vi "Configure Hardware.vi"(8 "error in (no error)":T3 caption="entrée d'erreur (pas d'erreur)", 11 "Ressources matérielles en entrée":T1) -> (0 "error out":T3 caption="sortie d'erreur", 3 "Ressources matérielles en sortie":T1)   [LabVIEW 2020, in "Acquisition.lvlib"]
doc: "Configurez le matériel."
uses:
  Acquisition.lvlib
  Hardware Configuration.ctl
  Signal Type.ctl
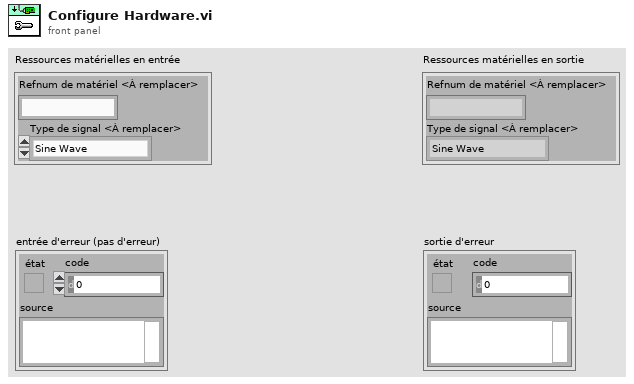
[diagram p1: front panel]
types:
  T1 = typedef "Acquisition.lvlib/Hardware Configuration.ctl" = cluster{"Refnum de matériel <À remplacer>":string, "Type de signal <À remplacer>":T2}
  T2 = typedef "Acquisition.lvlib/Signal Type.ctl" = enum16{"Sine Wave", "Square with Noise", "Signal triangulaire", "Simulation DAQ"}
  T3 = cluster{"état":bool, "code":i32, "source":string}
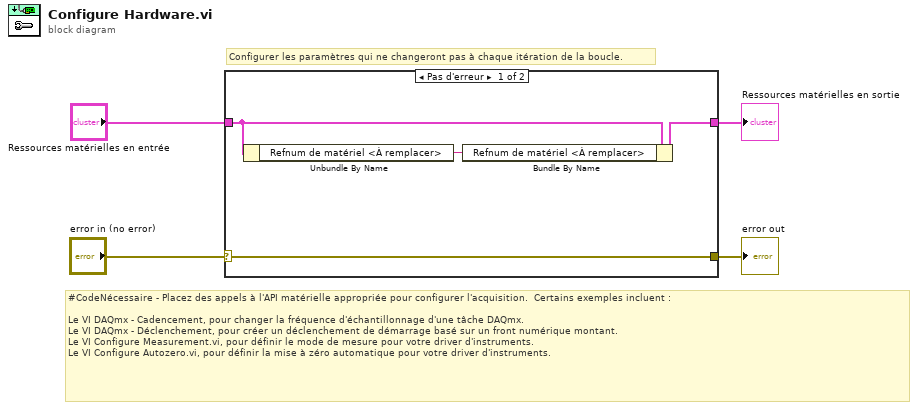
[diagram p0: block diagram]
diagram:
  # "Configurer les paramètres qui ne changeront pas à chaque itération de la boucle."
  # "#CodeNécessaire - Placez des appels à l'API matérielle appropriée pour configurer l'acquisition.  Certains exemples incluent :\n\nLe VI DAQmx - Cadencement, pour changer la fréquence d'échantillonnage d'une tâche DAQmx.\nLe VI DAQmx - Déclenchement, pour créer un déclenchement de démarrage basé sur un front numérique montant.\nLe VI Configure Measurement.vi, pour définir le mode de mesure pour votre driver d'instruments.\nLe VI Configure Autozero.vi, pour définir la mise à zéro automatique pour votre driver d'instruments."
  n1 = case shown="Pas d'erreur" "error in (no error)" {
    selector: "error in (no error)" -> [w7 w9]
    tunnel: [w7 w9] -> w3
    tunnel: "Ressources matérielles en entrée" -> [w6 w10]
    tunnel: [w8 w10] -> w1
    frame No Error {
      n2 = Unbundle By Name(w6) -> ("Refnum de matériel <À remplacer>"=w5:string)
      n3 = Bundle By Name(cluster=w6, "Refnum de matériel <À remplacer>"=w5) -> (w8:T1)
    }
    frame Error {
    }
  }
  "Ressources matérielles en sortie" <- w1
  "error out" <- w3
